vi "NumIntegrate_Rk4_Dbl_X_U.vi"(7 "ExtraData":variant, 8 "DT":dbl, 10 "U":dbl, 11 "X":dbl) -> (3 "Integral":dbl)   [LabVIEW 2019, in "Trajectory_Library.lvlib"]
doc: "NOT DONE"
uses:
  Trajectory_Library.lvlib
panel:
  in  "Func":refnum<vi>
  out "Error":bool
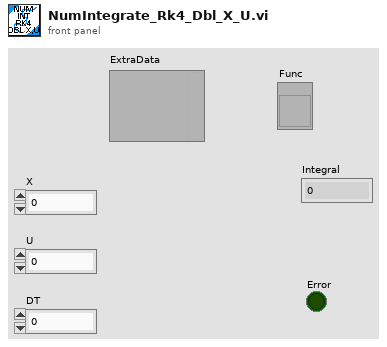
[diagram p1: front panel]
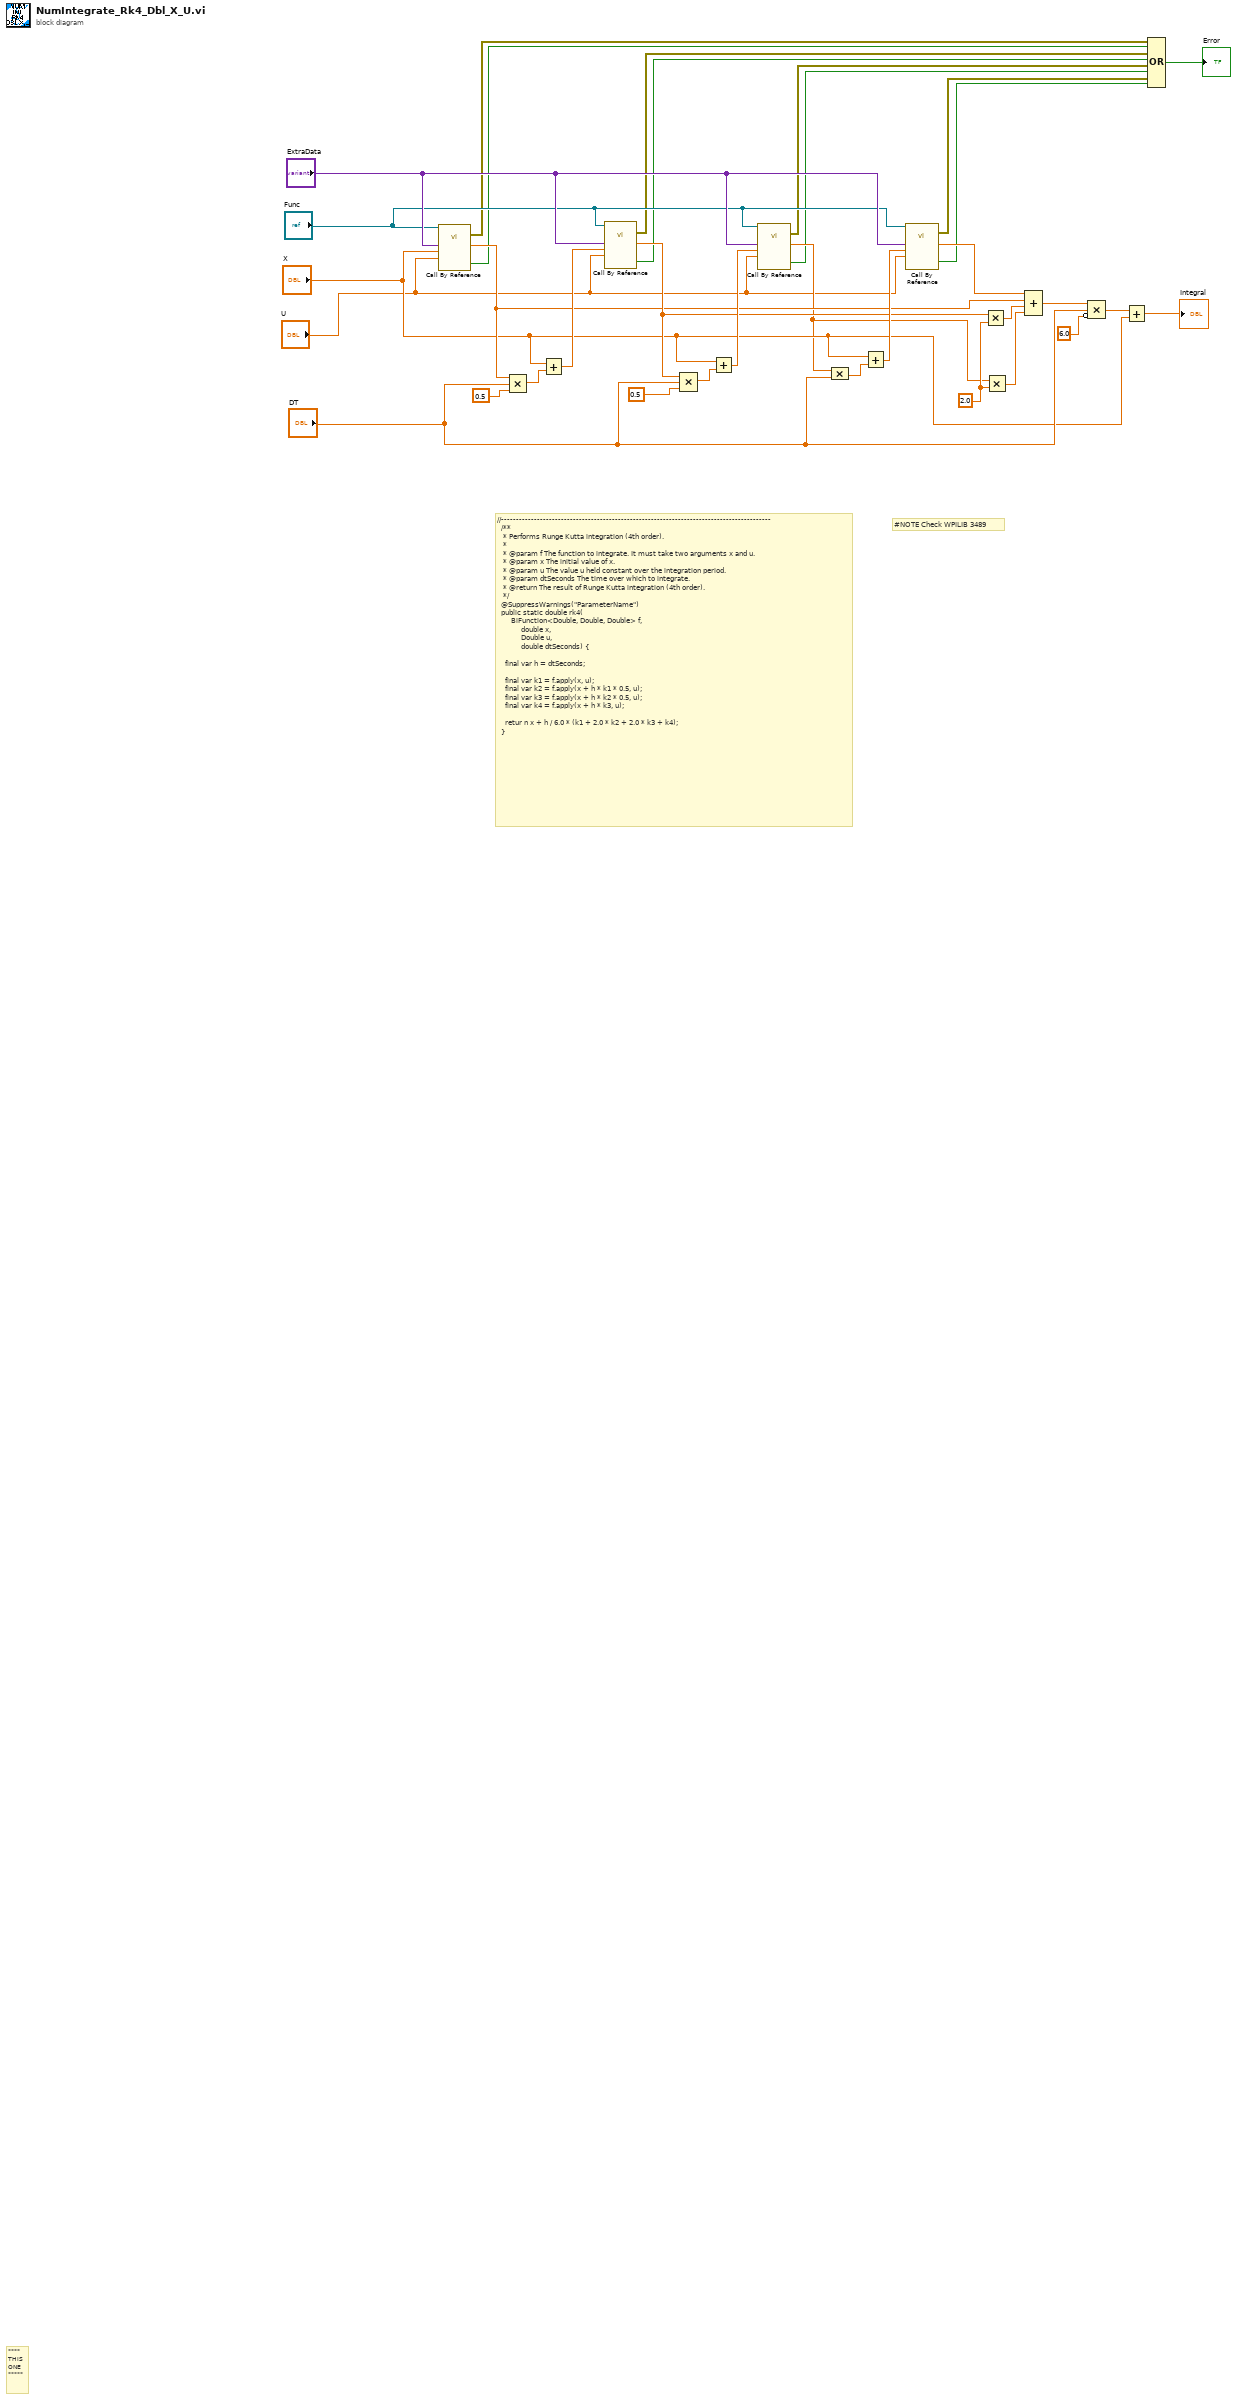
[diagram p0: block diagram]
diagram:
  w21 = 2.0 ("y")
  # "#NOTE Check WPILIB 3489"
  # "//------------------------------------------------------------------------------------------\n  /**\n   * Performs Runge Kutta integration (4th order).\n   *\n   * @param f The function to integrate. It must take two arguments x and u.\n   * @param x The initial value of x.\n   * @param u The value u held constant over the integration period.\n   * @param dtSeconds The time over which to integrate.\n   * @return The result of Runge Kutta integration (4th order).\n   */\n  @SuppressWarnings(\"ParameterName\")\n  public static double rk4(\n      \tBiFunction<Double, Double, Double> f, \n           \tdouble x, \n\t           Double u, \n\t           double dtSeconds) {\n\n    final var h = dtSeconds;\n\n    final var k1 = f.apply(x, u);\n    final var k2 = f.apply(x + h * k1 * 0.5, u);\n    final var k3 = f.apply(x + h * k2 * 0.5, u);\n    final var k4 = f.apply(x + h * k3, u);\n\n    retur n x + h / 6.0 * (k1 + 2.0 * k2 + 2.0 * k3 + k4);\n  }"
  # "****\nTHIS\nONE\n*****"
  n1 = call-by-ref "?"(reference="Func", "U"="U", "X"="X", "Variant"="ExtraData") -> (error out=w8:errorcluster, "Error"=w7:bool, "NewX"=w23:dbl)  [unwired: 8 in, 1 out]
  n2 = Compound Arithmetic op=MULTIPLY(w23, "DT", 0.5 ("value")) -> (w32:dbl)
  n3 = Add(x="X", y=w32) -> (x+y=w31:dbl)
  n4 = call-by-ref "?"(reference="Func", "U"="U", "X"=w31, "Variant"="ExtraData") -> (error out=w6:errorcluster, "Error"=w5:bool, "NewX"=w24:dbl)  [unwired: 8 in, 1 out]
  n5 = Compound Arithmetic op=MULTIPLY(w24, "DT", 0.5 ("value")) -> (w29:dbl)
  n6 = Add(x="X", y=w29) -> (x+y=w28:dbl)
  n7 = call-by-ref "?"(reference="Func", "U"="U", "X"=w28, "Variant"="ExtraData") -> (error out=w4:errorcluster, "Error"=w3:bool, "NewX"=w12:dbl)  [unwired: 8 in, 1 out]
  n8 = Compound Arithmetic op=MULTIPLY(w12, "DT") -> (w26:dbl)
  n9 = Add(x="X", y=w26) -> (x+y=w25:dbl)
  n10 = call-by-ref "?"(reference="Func", "U"="U", "X"=w25, "Variant"="ExtraData") -> (error out=w2:errorcluster, "Error"=w1:bool, "NewX"=w22:dbl)  [unwired: 8 in, 1 out]
  n11 = Multiply(x=w24, y=w21) -> (x*y=w20:dbl)
  n12 = Multiply(x=w12, y=w21) -> (x*y=w19:dbl)
  n13 = Compound Arithmetic op=ADD(w22, w23, w20, w19) -> (w18:dbl)
  n14 = Compound Arithmetic op=MULTIPLY(w18, "DT", invert 6.0 ("y")) -> (w15:dbl)
  n15 = Add(x=w15, y="X") -> (x+y=→"Integral":dbl)
  n16 = Compound Arithmetic op=OR(w8, w7, w6, w5, w4, w3, w2, w1) -> (→"Error":bool)
